vi "Receiver_32.vi"() -> ()   [LabVIEW 2015]
uses:
  <vilib>/measure/matone.llb/Extract Single Tone Information 1 Chan.vi
  <vilib>/measure/NI_MAPro.lvlib
panel:
  out "full wave":dbl(graph)
  out "DE":i32(graph)
  out "detected amplitude":dbl format="%.2p"
  in  "Numeric":i32
  out "Output Chart":dbl(graph)
  out "Modulating Square Chart":i8(graph)
  in  "Number of Cycles":i32
  in  "number of bits":dbl
  out "Modulating Square":i8[](graph)
  out "Carrier":dbl[](graph)
  out "output":dbl[](graph)
  in  "Carrier Frequency":i32
  in  "Sampling freq.":i32
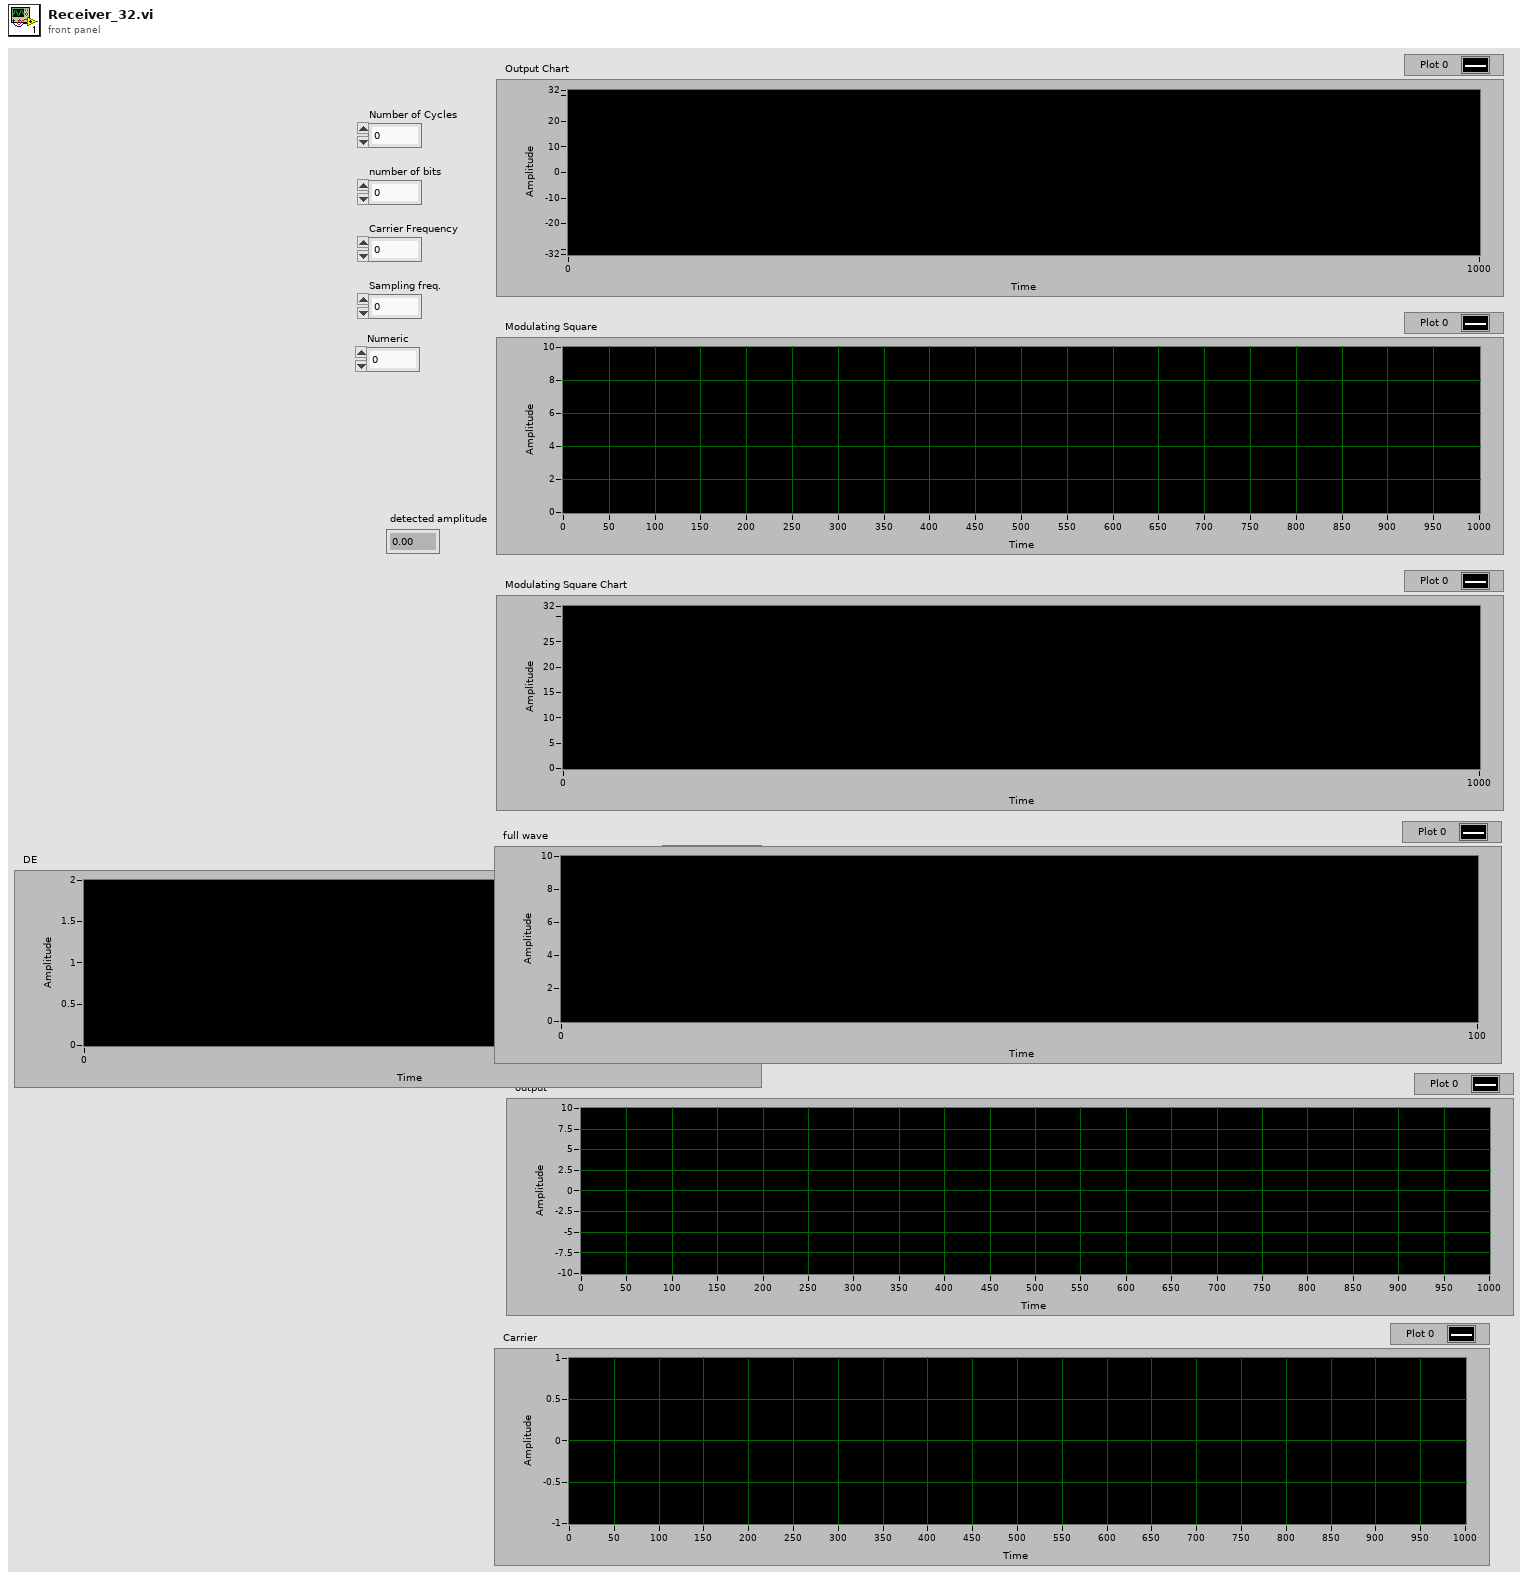
[diagram p1: front panel]
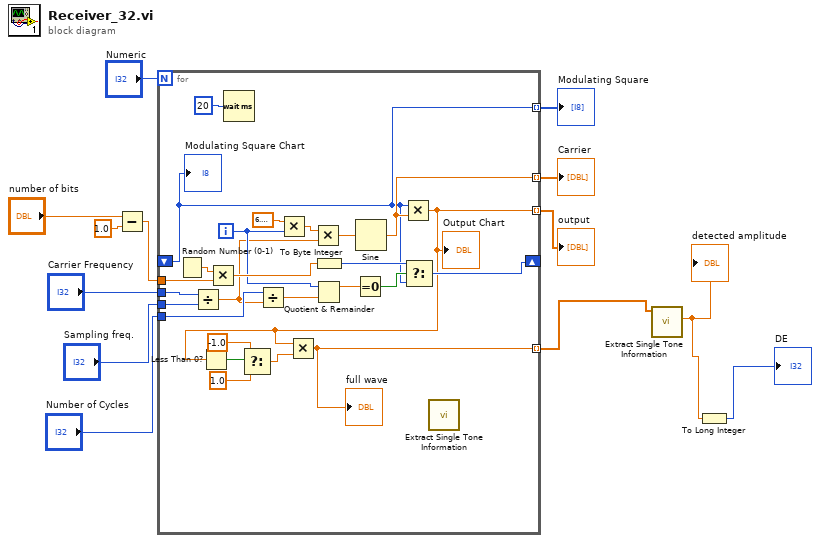
[diagram p0: block diagram]
diagram:
  n1 = Subtract(x="number of bits", y=1.0) -> (x-y=w6:dbl)
  n2 = for {
    N: "Numeric" -> [_]
    tunnel: "Sampling freq." -> [w38]
    tunnel: "Carrier Frequency" -> [w26]
    tunnel: [w16] -> w4 mode=indexing
    tunnel: [w36] -> w11 mode=indexing
    tunnel: w6 -> [w34]
    shift-right: [w28] -> _
    shift-left: _ -> [w20]
    tunnel: "Number of Cycles" -> [w24]
    tunnel: [w20] -> w13 mode=indexing
    tunnel: [w14] -> w3 mode=indexing
    i -> [w25]
    n3 = Random Number (0-1)() -> (number: 0 to 1=w35:dbl)
    n4 = Divide(x=w26, y=w38) -> (x/y=w23:dbl)
    n5 = Multiply(x=w35, y=w34) -> (x*y=w33:dbl)
    n6 = Wait (ms)(milliseconds to wait=u32 20) -> ()  [unwired: 1 out]
    n7 = Divide(x=w24, y=w23) -> (x/y=w22:dbl)
    n8 = Multiply(x=6.283185307179586, y=w25) -> (x*y=w32:dbl)
    n9 = Multiply(x=w32, y=w23) -> (x*y=w37:dbl)
    n10 = To Byte Integer(number=w33) -> (8bit integer=w29:i8)
    n11 = Quotient & Remainder(x=w25, y=w22) -> (x-y*floor(x/y)=w31:dbl)  [unwired: 1 out]
    n12 = Equal To 0?(x=w31) -> (x = 0?=w30:bool)
    n13 = Sine(x=w37) -> (sin(x)=w36:dbl)
    n14 = Multiply(x=w20, y=w36) -> (x*y=w16:dbl)
    "Output Chart" <- w16
    n15 = Less Than 0?(x=w16) -> (x < 0?=w19:bool)
    n16 = Select(t=-1.0, s=w19, f=1.0) -> (s? t:f=w15:dbl)
    n17 = Multiply(x=w16, y=w15) -> (x*y=w14:dbl)
    "full wave" <- w14
    n18 = Select(t=w29, s=w30, f=w20) -> (s? t:f=w28:i8)
    n19 = call-poly <vilib>:"Extract Single Tone Information.vi"() -> ()  [unwired: 6 in, 6 out]
    "Modulating Square Chart" <- w20
  }
  "output" <- w4
  "Carrier" <- w11
  "Modulating Square" <- w13
  n20 = call-poly <vilib>:"Extract Single Tone Information.vi"("time signal in"=w3) -> ("detected amplitude"=w2:dbl)  [unwired: 5 in, 5 out]
  "detected amplitude" <- w2
  n21 = To Long Integer(number=w2) -> (32bit integer=→"DE":i32)
